vi "Test_Lockin_API.vi"() -> ()   [LabVIEW 2016]
uses:
  RemoteControl/Typedefs/Remote-SMO-Commands-Enum.ctl
  Typedefs/AO-cluster.ctl
  Typedefs/AO_Amp-array.ctl
  Typedefs/AO_DC-array.ctl
  Typedefs/AO_f-array.ctl
  Typedefs/AO_phi-array.ctl
  Typedefs/Function-array.ctl
  Typedefs/Function-enum.ctl
  Typedefs/REF-cluster.ctl
  Typedefs/REF_f-array.ctl
  Typedefs/REF_phi-array.ctl
  RemoteControl/RemoteControl.lvclass
panel:
  in  "Tab Control":enum32{"getResults", "getAO", "getAI", "config"}(tab)
  out "getResults":dbl(graph)
  in  "disabled index (col)":i32
  in  "disabled index (row)":i32
  out "getAO":waveform(dbl)[](graph)
  out "getAI":waveform(dbl)[](graph)
  in  "Channels: AO":T1 {"AO f (Hz)" min=0.001 max=10000.0; "AO DC (V)" format="%#_6p"; "AO amp (V)" format="%#_6p"}
  in  "Channels: Lockin":T8 {"REF phi (deg)" format="%#_3g"}
  in  "IV mode":bool
  in  "Remote Mode":bool=TRUE
  in  "Trigger":bool=TRUE
  out "ms watiing for IV curve":u32
  out "Numeric":i32
  in  "address":string
  in  "Enum":T11
  in  "Stop":bool
  # "0"
  # "1"
  # "2"
  # "3"
  # "4"
  # "5"
  # "6"
  # "7"
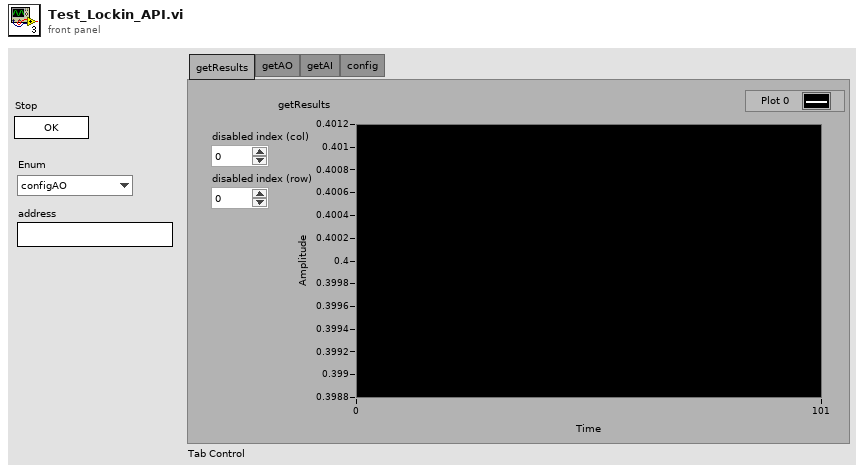
[diagram p1: front panel]
types:
  T1 = typedef "AO-cluster.ctl" = cluster{"AO amp (V)":T2, "AO DC (V)":T3, "AO f (Hz)":T4, "AO phi (deg)":T5, "function":T6}
  T2 = typedef "AO_Amp-array.ctl" = dbl[]
  T3 = typedef "AO_DC-array.ctl" = dbl[]
  T4 = typedef "AO_f-array.ctl" = dbl[]
  T5 = typedef "AO_phi-array.ctl" = dbl[]
  T6 = typedef "Function-array.ctl" = T7[]
  T7 = typedef "Function-enum.ctl" = enum16{"Sine Wave", "Triangle Wave", "Square Wave", "Sawtooth Wave"}
  T8 = typedef "REF-cluster.ctl" = cluster{"REF f (Hz)":T9, "REF phi (deg)":T10}
  T9 = typedef "REF_f-array.ctl" = dbl[]
  T10 = typedef "REF_phi-array.ctl" = dbl[]
  T11 = typedef "RemoteControl.lvclass/Remote-SMO-Commands-Enum.ctl" = enum16{"configAO", "configREF", "configIVmode", "configRemote", "assertTrigger", "getAO", "getAI", "getResults", "getTrigger", "getAOconfig", "getREFconfig", "ACK", "UNK", "CLOSE"}
  T12 = enum32{"invalid app kind", "Development System", "Run Time System", "Student Edition", "Embedded LabVIEW", "Evaluation", "Custom"}
  T13 = enum32{"Invalid", "Standard", "Closed", "Hidden", "Minimized", "Maximized"}
  T14 = cluster{"Core":cluster{"Current VI Reference":refnum<vi>, "Close Panel on Exit?":bool}, "Your Boolean data":bool, "remote address":string}
  T15 = cluster{"Current VI Reference":refnum<vi>, "Close Panel on Exit?":bool}
  T16 = typedef "RemoteControl.lvclass/PrivateEvents--RemoteControl.setTrigger.ctl" = bool
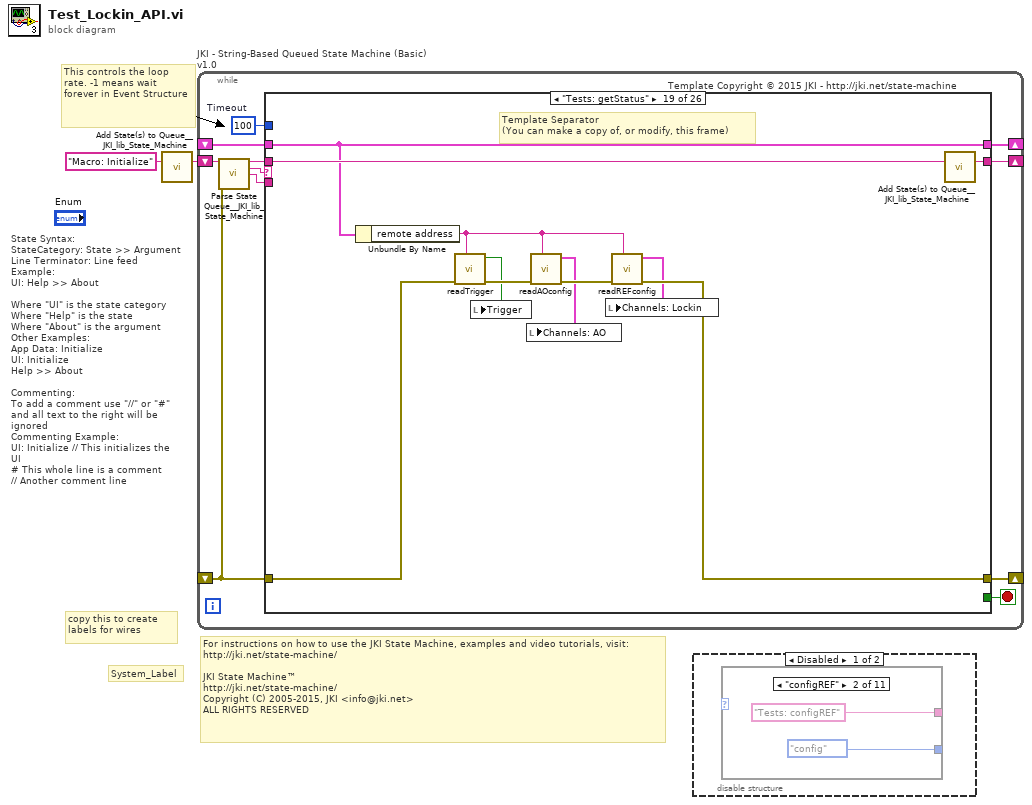
[diagram p0: block diagram]
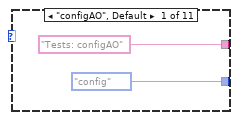
[diagram p2: hidden frame]
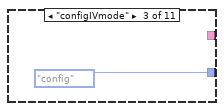
[diagram p3: hidden frame]
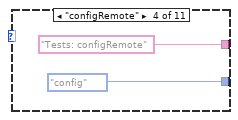
[diagram p4: hidden frame]
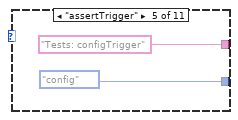
[diagram p5: hidden frame]
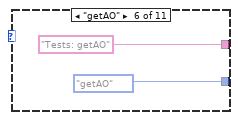
[diagram p6: hidden frame]
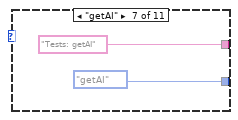
[diagram p7: hidden frame]
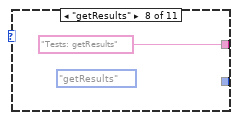
[diagram p8: hidden frame]
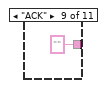
[diagram p9: hidden frame]
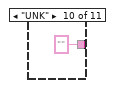
[diagram p10: hidden frame]
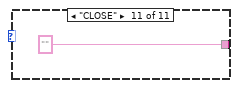
[diagram p11: hidden frame]
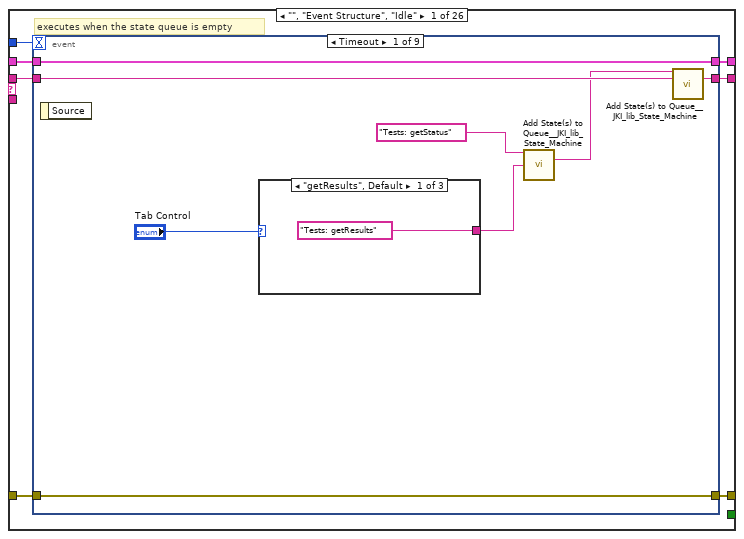
[diagram p13: hidden frame]
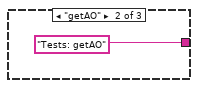
[diagram p14: hidden frame]
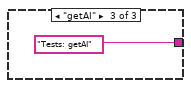
[diagram p15: hidden frame]
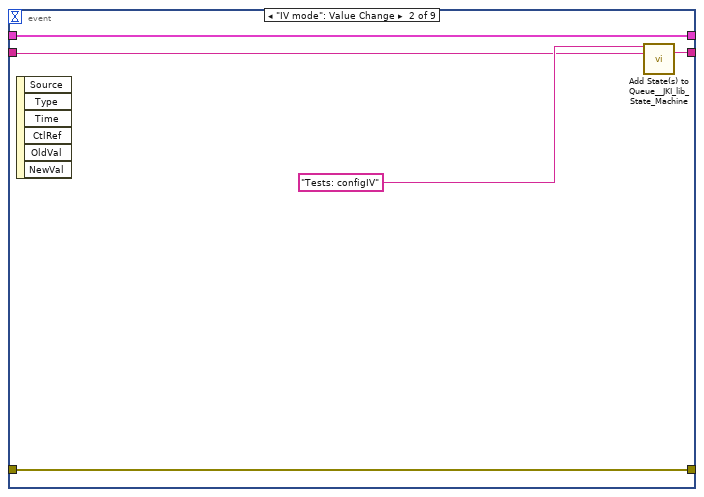
[diagram p16: hidden frame]
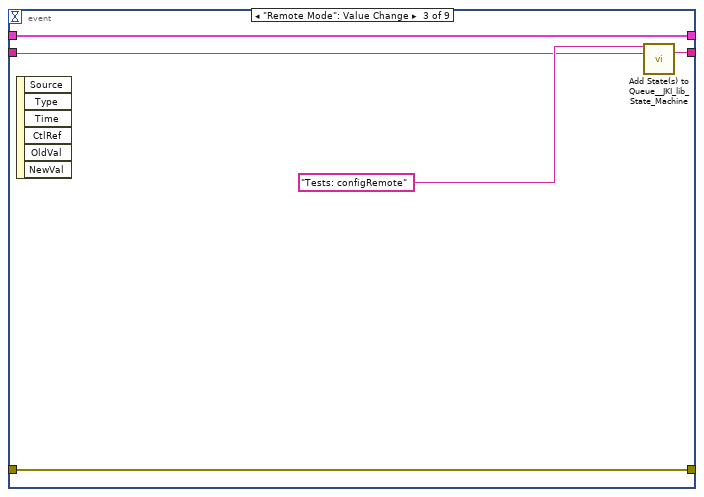
[diagram p17: hidden frame]
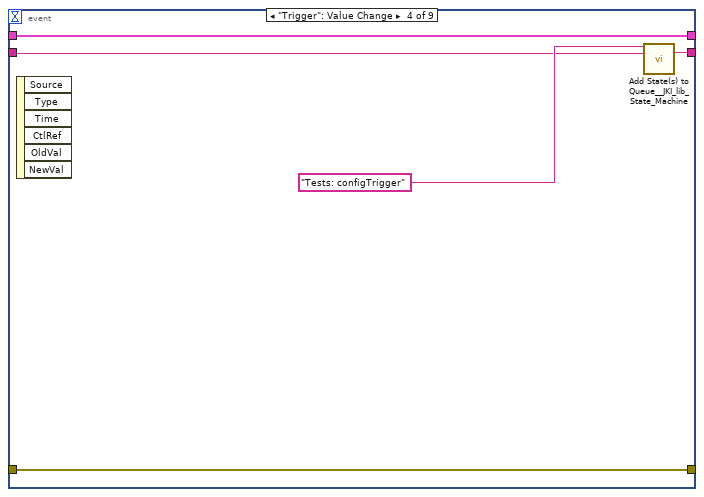
[diagram p18: hidden frame]
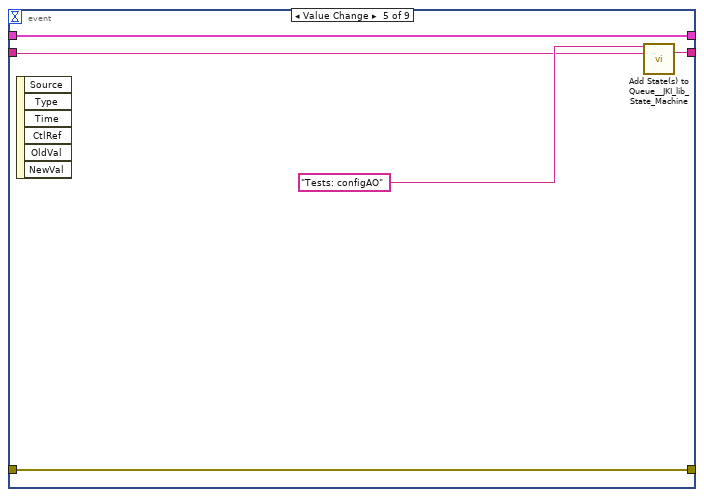
[diagram p19: hidden frame]
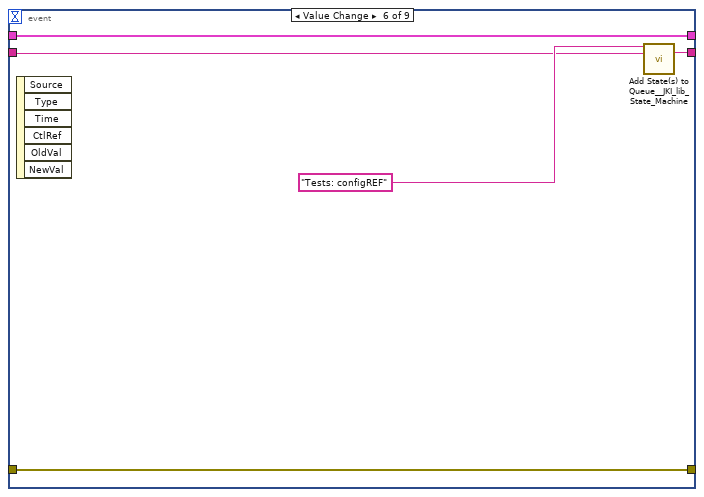
[diagram p20: hidden frame]
diagram:
  # "For instructions on how to use the JKI State Machine, examples and video tutorials, visit:\nhttp://jki.net/state-machine/\n\nJKI State Machine™\nhttp://jki.net/state-machine/\nCopyright (C) 2005-2015, JKI <info@jki.net>\nALL RIGHTS RESERVED"
  # "State Syntax:\nStateCategory: State >> Argument\nLine Terminator: Line feed\nExample:\nUI: Help >> About\n\nWhere \"UI\" is the state category\nWhere \"Help\" is the state\nWhere \"About\" is the argument\nOther Examples:\nApp Data: Initialize\nUI: Initialize\nHelp >> About\n\nCommenting:\nTo add a comment use \"//\" or \"#\" and all text to the right will be ignored\nCommenting Example:\nUI: Initialize // This initializes the UI\n# This whole line is a comment\n// Another comment line"
  # "copy this to create labels for wires"
  # "This controls the loop rate. -1 means wait forever in Event Structure"
  # "System_Label"
  n1 = call <vilib>:"Add State(s) to Queue__JKI_lib_State_Machine.vi"("State(s) in (\"\")"="Macro: Initialize") -> ("States Out"=w2:string)  [unwired: 14 in]
  n2 = while "JKI - String-Based Queued State Machine (Basic) v1.0" {
    shift-right: [w6] -> _
    shift-left: _ -> [w5]
    shift-right: [w9] -> _
    shift-left: _ -> [w3]
    shift-right: [w8] -> _
    shift-left: w2 -> [w10]
    stop <- w7 stop-if-true
    w4 = 100  # Timeout
    # "Template Copyright © 2015 JKI - http://jki.net/state-machine"
    n3 = call <vilib>:"Parse State Queue__JKI_lib_State_Machine.vi"("State Queue"=w10, "Error In (no error)"=w3) -> ("Remaining States"=w12:string, "Current State"=w13:string, "Arguments"=w11:string)  [unwired: 11 in]
    n4 = case shown="\"Tests: getStatus\"" w13 {
      selector: w13 -> [_ _ w78 _ _ _ _ _ _ _ _ _ _ _ _ _ _ _ _ _ _ _ _ _ _ _]
      tunnel: w12 -> [w20 w77 w82 w100 w106 w111 w115 w122 w128 w132 w136 w142 w153 w179 w184 w194 w198 w208 w219 w226 w233 w240 w247 w254 w261 w271]
      tunnel: w11 -> [_ _ _ _ _ _ _ _ _ _ _ w137 w147 _ _ _ _ _ _ _ _ _ _ _ _ _]
      tunnel: w5 -> [w18 w74 w80 w91 w103 w109 w112 _ w123 w129 w134 w140 w149 w176 w181 w191 w195 w200 w217 w220 w227 w234 w241 w248 w255 w266]
      tunnel: [w17 w75 w84 w97 errorcluster {"status"=FALSE, "code"=0, "source"=""} ("error out") w108 w113 w119 w124 w130 w133 w138 w150 w177 w182 w192 w196 w201 w212 w222 w230 w236 w243 w251 w258 w265] -> w9
      tunnel: w3 -> [w16 w75 w83 w97 w102 w108 w113 w119 w125 w130 w133 w139 w151 w177 w182 w192 w196 w202 w213 w224 w231 w237 w244 w252 w259 w269]
      tunnel: [w19 w76 w81 w99 w105 w110 w114 w121 w127 w131 w135 w141 w152 w178 w183 w193 w197 w207 w218 w225 w232 w239 w246 w253 w260 w270] -> w8
      tunnel: [_ _ _ _ _ TRUE _ _ _ _ _ _ _ _ _ _ _ _ _ _ _ _ _ _ _ _] -> w7
      tunnel: [w15 w74 w80 w98 w103 w109 w112 w120 w123 w129 w134 w140 w149 w176 w181 w191 w195 w200 w217 w220 w227 w234 w241 w248 w255 w266] -> w6
      tunnel: w4 -> [w14 _ _ _ _ _ _ _ _ _ _ _ _ _ _ _ _ _ _ _ _ _ _ _ _ _]
      frame "", "Event Structure", "Idle" {
        # "executes when the state queue is empty"
        n5 = event shown="[0] Timeout" {
          selector: _ -> [_ _ _ _ _ _ _ _ _]
          dyn-events: _ -> [_ _ _ _ _ _ _ _ _]
          timeout: w14 -> [_ _ _ _ _ _ _ _ _]
          tunnel: w20 -> [w28 w32 w37 w42 w47 w52 w61 w67 w73]
          tunnel: [w27 w36 w41 w46 w51 w56 w62 w66 w72] -> w19
          tunnel: w18 -> [w26 w33 w38 w43 w48 w53 w59 w64 w70]
          tunnel: [w24 w34 w39 w44 w49 w54 w60 w65 w71] -> w17
          tunnel: w16 -> [w24 w34 w39 w44 w49 w54 w60 w65 w71]
          tunnel: [w26 w33 w38 w43 w48 w53 w58 w64 w70] -> w15
          event Timeout {
            n6 = event-data() -> ()  [unwired: 1 in, 1 out]
            n7 = case shown="\"getResults\", Default" "Tab Control" {
              tunnel: ["Tests: getResults" "Tests: getAO" "Tests: getAI"] -> w23
              frame "getResults", Default {
              }
              frame "getAO" {
              }
              frame "getAI" {
              }
            }
            n8 = call <vilib>:"Add State(s) to Queue__JKI_lib_State_Machine.vi"("State(s) in Front (\"\")"="Tests: getStatus", "State(s) at Back (\"\")"=w23) -> ("States Out"=w22:string)  [unwired: 13 in]
            n9 = call <vilib>:"Add State(s) to Queue__JKI_lib_State_Machine.vi"("State(s) in Front (\"\")"=w22, "State(s) in (\"\")"=w28) -> ("States Out"=w27:string)  [unwired: 13 in]
          }
          event "IV mode": Value Change {
            n10 = event-data() -> ()  [unwired: 1 in, 6 out]
            n11 = call <vilib>:"Add State(s) to Queue__JKI_lib_State_Machine.vi"("State(s) in Front (\"\")"="Tests: configIV", "State(s) in (\"\")"=w32) -> ("States Out"=w36:string)  [unwired: 13 in]
          }
          event "Remote Mode": Value Change {
            n12 = event-data() -> ()  [unwired: 1 in, 6 out]
            n13 = call <vilib>:"Add State(s) to Queue__JKI_lib_State_Machine.vi"("State(s) in Front (\"\")"="Tests: configRemote", "State(s) in (\"\")"=w37) -> ("States Out"=w41:string)  [unwired: 13 in]
          }
          event "Trigger": Value Change {
            n14 = event-data() -> ()  [unwired: 1 in, 6 out]
            n15 = call <vilib>:"Add State(s) to Queue__JKI_lib_State_Machine.vi"("State(s) in Front (\"\")"="Tests: configTrigger", "State(s) in (\"\")"=w42) -> ("States Out"=w46:string)  [unwired: 13 in]
          }
          event Value Change {
            n16 = event-data() -> ()  [unwired: 1 in, 6 out]
            n17 = call <vilib>:"Add State(s) to Queue__JKI_lib_State_Machine.vi"("State(s) in Front (\"\")"="Tests: configAO", "State(s) in (\"\")"=w47) -> ("States Out"=w51:string)  [unwired: 13 in]
          }
          event Value Change {
            n18 = event-data() -> ()  [unwired: 1 in, 6 out]
            n19 = call <vilib>:"Add State(s) to Queue__JKI_lib_State_Machine.vi"("State(s) in Front (\"\")"="Tests: configREF", "State(s) in (\"\")"=w52) -> ("States Out"=w56:string)  [unwired: 13 in]
          }
          event "address": Value Change {
            n20 = event-data() -> ()  [unwired: 1 in, 6 out]
            n21 = Bundle By Name(cluster=w59, "remote address"="address") -> (w58:T14)
            n22 = call <vilib>:"Add State(s) to Queue__JKI_lib_State_Machine.vi"("State(s) in (\"\")"=w61) -> ("States Out"=w62:string)  [unwired: 14 in]
          }
          event "Stop": Value Change {
            # "Exit Button Value Change (pressed) Event\n(this executes Macro: Exit to terminate the VI)"
            n23 = event-data() -> ()  [unwired: 1 in, 1 out]
            n24 = call <vilib>:"Add State(s) to Queue__JKI_lib_State_Machine.vi"("State(s) in Front (\"\")"="Macro: Exit", "State(s) in (\"\")"=w67) -> ("States Out"=w66:string)  [unwired: 13 in]
          }
          event Panel Close? {
            # "Discard the event because we'll close the front panel ourselves in Macro: Exit"
            # "Close Panel button (pressed) Event\n(this executes Macro: Exit to terminate the VI)"
            n25 = event-data() -> ()  [unwired: 1 in, 1 out]
            n26 = event-data("Discard?"=TRUE) -> ()  [unwired: 1 in, 1 out]
            n27 = call <vilib>:"Add State(s) to Queue__JKI_lib_State_Machine.vi"("State(s) in Front (\"\")"="Macro: Exit", "State(s) in (\"\")"=w73) -> ("States Out"=w72:string)  [unwired: 13 in]
          }
        }
      }
      frame "---------- Core ----------" {
        # "Do not put any code in this frame.\n(it is a separator no-op)"
        n28 = call <vilib>:"Add State(s) to Queue__JKI_lib_State_Machine.vi"("State(s) in (\"\")"=w77) -> ("States Out"=w76:string)  [unwired: 14 in]
      }
      frame Default {
        w87 = 42 items=["No error", "Argument error", "Memory is full", "Out of zone", "End of file", "File already open", "Generic file I/O error", "File not found", "File permission error", "Disk is full", "Duplicate path", "Too many files open", "System feature not enabled", "Resource file not found", "Cannot add resource", "Resource not found", "Image not found", "Image memory error", "Pen does not exist", "Config type invalid", "Config token not found", "Config parse error", "Config memory error", "Bad external code format", "Bad external code offset", "External code not present", "Null window", "Destroy window error", "Null menu", "Print aborted", "Bad print record", "Print driver error", "Windows error during printing", "Memory error during printing", "Print dialog error", "Generic print error", "Invalid device refnum", "Device not found", "Device parameter error", "Device unit error", "Cannot open device", "Device call aborted", "Generic error", "Cancelled by user", "Object ID too low", "Object ID too high", "Object not in heap", "Unknown heap", "Unknown object (invalid DefProc)", "Unknown object (DefProc not in table)", "Message out of range", "Invalid (null) method", "Unknown message", "Manager call not supported", "Bad address", "Network operation in progress", "Network operation timed out", "Connection is busy", "Network attribute not supported", "Network error", "Address in use", "System out of memory", "Connection aborted", "Connection refused", "Not connected", "Already connected", "Connection closed", "Initialization error (interapplication manager)", "Bad occurrence", "Wait on unbound occurrence handler", "Occurrence queue overflow", "Datalog type conflict", "Unused", "Unrecognized type (interapplication manager)", "Memory corrupt", "Failed to make temporary DLL", "Old CIN version", "Drag socket not found", "Failed to load drop-object", "Failed to register OLE object", "Failed to release OLE object", "Format specifier type mismatch", "Unknown format specifier", "Too few format specifiers", "Too many format specifiers", "Scan failed", "Newer CIN version", "Error converting to variant", "Runtime menu error", "Password tampered", "Variant attribute not found", "Incompatible variant data type", "Event data is not available", "Event Store is not present", "Occurrence is not found", "Event Queue is not created", "Event info is not available", "Refnum passed is NULL", "Error retrieving Class GUID", "Error retrieving CoClass GUID", "Error retrieving TypeLib GUID.", "Bad built application magic bytes.", "Specific driver is different from the specific driver associated with the Logical Name.", "There is no session opened to the class driver.", "Max Error", "MAX - Error with config objects", "MAX - Error loading configuration", "MAX - Group not supported"]
        # "Current State"
        # "Do not delete, rename, or modify this frame.\n(this is used to capture unhandled states and typos)"
        # "Handle mistyped state name (developer tool)"
        n29 = Format Into String(format string="Software Exception: Unhandled State \"%s\"." ("message"), error in=w83, w78) -> (resulting string=w86:string, error out=w85:errorcluster)  [unwired: 1 in]
        n30 = call <vilib>:"Error Cluster From Error Code.vi"("show call chain? (False)"=TRUE, "error in (no error)"=w85, "error message (\"\")"=w86, "error code (0)"=w87) -> ("error out"=w84:errorcluster)  [unwired: 5 in]
        n31 = call <vilib>:"Add State(s) to Queue__JKI_lib_State_Machine.vi"("State(s) in (\"\")"=w82) -> ("States Out"=w81:string)  [unwired: 14 in]
      }
      frame "Initialize Core Data" {
        # "Do not delete, rename, or modify this frame.\n(this is used to determine panel behavior on exit)"
        # "originally closed?"
        # "exe?"
        # "If panel starts closed or is an EXE, then close it when we exit"
        n32 = property class="VI"() -> ("Front Panel.Open"=w96:bool)  [unwired: 2 in, 2 out]
        n33 = property class="App"() -> ("App.Kind"=w95:T12)  [unwired: 2 in, 2 out]
        n34 = control-ref of="Current VI Reference"() -> (w89:refnum<vi>)
        n35 = Not(x=w96) -> (.not. x?=w93:bool)
        n36 = Equal?(x=w95, y=T12."Run Time System" ("Application:Kind")) -> (x = y?=w92:bool)
        n37 = Or(x=w93, y=w92) -> (x .or. y?=w90:bool)
        n38 = Bundle By Name(cluster=w91, "Core.Current VI Reference"=w89, "Core.Close Panel on Exit?"=w90) -> (w98:T14)
        n39 = call <vilib>:"Add State(s) to Queue__JKI_lib_State_Machine.vi"("State(s) in (\"\")"=w100) -> ("States Out"=w99:string)  [unwired: 14 in]
      }
      frame "Error Handler" {
        # "Unhandled Error -- Display it"
        # "Handle any errors here.\nYou can also output any states to clean-up after errors occur"
        # "Clear error"
        n40 = call <vilib>:"General Error Handler.vi"("error in (no error)"=w102) -> ()  [unwired: 10 in, 5 out]
        n41 = call <vilib>:"Add State(s) to Queue__JKI_lib_State_Machine.vi"("State(s) in Front (\"\")"="/* Post Error States", "State(s) in (\"\")"=w106) -> ("States Out"=w105:string)  [unwired: 13 in]
      }
      frame "Exit" {
        # "Do not put any code in this frame.\n(No errors that occur here will be handled.)"
        n42 = call <vilib>:"Add State(s) to Queue__JKI_lib_State_Machine.vi"("State(s) in (\"\")"=w111) -> ("States Out"=w110:string)  [unwired: 14 in]
      }
      frame "---------- Data ----------" {
        # "Do not put any code in this frame.\n(It is a separator no-op. You can make a copy of this frame to create a new Data frame)"
        n43 = call <vilib>:"Add State(s) to Queue__JKI_lib_State_Machine.vi"("State(s) in (\"\")"=w115) -> ("States Out"=w114:string)  [unwired: 14 in]
      }
      frame "Data: Initialize" {
        w116 = T15 {"Current VI Reference"=refnum, "Close Panel on Exit?"=FALSE}  # Core
        w118 = TRUE  # Your Boolean data
        w117 = ""  # remote address
        # "do not delete - used by framework"
        # "Expand Bundle to add new data elements to shift register data."
        # "Data names and types of shift register data are defined by this bundle."
        # "Initialize the shift-register data, here.\n(data names are defined by what you wire into the bundle function)"
        n44 = Bundle("Core"=w116, "Your Boolean data"=w118, "remote address"=w117) -> (w120:T14)  [unwired: 1 in]
        n45 = call <vilib>:"Add State(s) to Queue__JKI_lib_State_Machine.vi"("State(s) in (\"\")"=w122) -> ("States Out"=w121:string)  [unwired: 14 in]
      }
      frame "Data: Cleanup" {
        # "Cleanup any data and references, here.\n(this is called automatically, by the Macro: Exit)"
        n46 = Unbundle By Name(w123) -> ("Core.Current VI Reference"=w126:refnum<vi>)
        n47 = Close Reference(reference=w126, error in (no error)=w125) -> (error out=w124:errorcluster)
        n48 = call <vilib>:"Add State(s) to Queue__JKI_lib_State_Machine.vi"("State(s) in (\"\")"=w128) -> ("States Out"=w127:string)  [unwired: 14 in]
      }
      frame "---------- UI ----------" {
        # "Do not put any code in this frame.\n(It is a separator no-op. You can make a copy of this frame to create a new UI frame)"
        n49 = call <vilib>:"Add State(s) to Queue__JKI_lib_State_Machine.vi"("State(s) in (\"\")"=w132) -> ("States Out"=w131:string)  [unwired: 14 in]
      }
      frame "UI: Initialize" {
        # "Initialize the User Interface, here.\n(this is called automatically, by the Macro: Init)"
        n50 = call <vilib>:"Add State(s) to Queue__JKI_lib_State_Machine.vi"("State(s) in (\"\")"=w136) -> ("States Out"=w135:string)  [unwired: 14 in]
      }
      frame "UI: Cursor Set" {
        # "Argument"
        # "Set and Unset Cursor Busy.\n(Usage: \"UI: Cursor Set >> Busy|Idle\")"
        n51 = case shown="\"Idle\", Default" w137 {
          tunnel: w139 -> [w144 w146]
          tunnel: [w143 w145] -> w138
          frame "Idle", Default {
            n52 = call <vilib>:"Unset Busy.vi"("error in (no error)"=w144) -> ("error out"=w143:errorcluster)  [unwired: 10 in]
          }
          frame "Busy" {
            n53 = call <vilib>:"Set Busy.vi"("error in (no error)"=w146) -> ("error out"=w145:errorcluster)  [unwired: 9 in, 1 out]
          }
        }
        n54 = call <vilib>:"Add State(s) to Queue__JKI_lib_State_Machine.vi"("State(s) in (\"\")"=w142) -> ("States Out"=w141:string)  [unwired: 14 in]
      }
      frame "UI: Front Panel State" {
        # "Argument"
        # "Set Front Panel Open or Closed\n(Usage: \"UI: Front Panel State >> Open|Close\")"
        n55 = Unbundle By Name(w149) -> ("Core.Current VI Reference"=w148:refnum<vi>)
        n56 = case shown="\"Open\", Default" w147 {
          tunnel: w151 -> [w157 w170]
          tunnel: [w159 w171] -> w150
          tunnel: w148 -> [w158 w168]
          frame "Open", Default {
            n57 = property class="VI"(reference=w158, error in=w157) -> (reference out=w155:refnum<vi>, error out=w156:errorcluster, "Front Panel.Open"=w154:bool)
            n58 = case shown="False" w154 {
              tunnel: [w162 w165] -> w159
              tunnel: w156 -> [w161 w165]
              tunnel: w155 -> [w160 _]
              frame False {
                n59 = invoke class="VI" method="FP.Open"(reference=w160, error in=w161, "Activate"=TRUE, "State"=T13."Standard") -> (error out=w162:errorcluster)  [unwired: 1 in, 4 out]
              }
              frame True {
              }
            }
          }
          frame "Close" {
            n60 = property class="VI"(reference=w168, error in=w170) -> (reference out=w167:refnum<vi>, error out=w169:errorcluster, "Front Panel.Open"=w166:bool)
            n61 = case shown="True" w166 {
              tunnel: [w172 w175] -> w171
              tunnel: w169 -> [w172 w174]
              tunnel: w167 -> [_ w173]
              frame False {
              }
              frame True {
                n62 = invoke class="VI" method="FP.Close"(reference=w173, error in=w174) -> (error out=w175:errorcluster)  [unwired: 1 in, 2 out]
              }
            }
          }
        }
        n63 = call <vilib>:"Add State(s) to Queue__JKI_lib_State_Machine.vi"("State(s) in (\"\")"=w153) -> ("States Out"=w152:string)  [unwired: 14 in]
      }
      frame "---------- Macro ----------" {
        # "Do not put any code in this frame.\n(It is a separator no-op. You can make a copy of this frame to create a new Macro frame)"
        n64 = call <vilib>:"Add State(s) to Queue__JKI_lib_State_Machine.vi"("State(s) in (\"\")"=w179) -> ("States Out"=w178:string)  [unwired: 14 in]
      }
      frame "Macro: Initialize" {
        w180 = "Data: Initialize\nInitialize Core Data\nUI: Initialize\nUI: Front Panel State >> Open"  # Data: Initialize Initialize Core Data UI: Initialize UI: Front Panel State >> Open
        # "Initialization Macro\n(This is called once, when the VI starts)"
        n65 = call <vilib>:"Add State(s) to Queue__JKI_lib_State_Machine.vi"("State(s) in Front (\"\")"=w180, "State(s) in (\"\")"=w184) -> ("States Out"=w183:string)  [unwired: 13 in]
      }
      frame "Macro: Exit" {
        # "Exit Macro\n(This is called once, when the VI exits)"
        n66 = Unbundle By Name(w191) -> ("Core.Close Panel on Exit?"=w190:bool)
        n67 = Select(t="UI: Front Panel State >> Close", s=w190, f="") -> (s? t:f=w187:string)
        n68 = call <vilib>:"Add State(s) to Queue__JKI_lib_State_Machine.vi"("State(s) in (\"\")"=w187, "State(s) at Back (\"\")"="Data: Cleanup\nExit") -> ("States Out"=w185:string)  [unwired: 13 in]
        n69 = call <vilib>:"Add State(s) to Queue__JKI_lib_State_Machine.vi"("State(s) in Front (\"\")"=w185, "State(s) in (\"\")"=w194) -> ("States Out"=w193:string)  [unwired: 13 in]
      }
      frame "---------- Tests ----------" {
        # "Template Separator\n(You can make a copy of, or modify, this frame)"
        n70 = call <vilib>:"Add State(s) to Queue__JKI_lib_State_Machine.vi"("State(s) in (\"\")"=w198) -> ("States Out"=w197:string)  [unwired: 14 in]
      }
      frame "Tests: getResults" {
        n71 = Unbundle By Name(w200) -> ("remote address"=w199:string)
        n72 = call "readResults.vi"("address"=w199, "error in (no error)"=w202) -> ("error out"=w201:errorcluster, "Results"=w203:dbl[][])  [unwired: 8 in]
        n73 = Index Array(array=w203, index (row)="disabled index (row)", index (col)="disabled index (col)") -> (element=→"getResults":dbl)
        n74 = call <vilib>:"Add State(s) to Queue__JKI_lib_State_Machine.vi"("State(s) in (\"\")"=w208) -> ("States Out"=w207:string)  [unwired: 14 in]
      }
      frame "Tests: getStatus" {
        # "Template Separator\n(You can make a copy of, or modify, this frame)"
        n75 = Unbundle By Name(w217) -> ("remote address"=w216:string)
        n76 = call "readTrigger.vi"("address"=w216, "error in (no error)"=w213) -> ("error out"=w215:errorcluster, "Trigger"=w209:T16)  [unwired: 8 in]
        n77 = local write "Trigger"(w209) -> ()
        n78 = call "readAOconfig.vi"("address"=w216, "error in (no error)"=w215) -> ("error out"=w214:errorcluster, "AOconfig"=w211:T1)  [unwired: 8 in]
        n79 = local write "Channels: AO"(w211) -> ()
        n80 = call "readREFconfig.vi"("address"=w216, "error in (no error)"=w214) -> ("error out"=w212:errorcluster, "REFconfig"=w210:T8)  [unwired: 8 in]
        n81 = local write "Channels: Lockin"(w210) -> ()
        n82 = call <vilib>:"Add State(s) to Queue__JKI_lib_State_Machine.vi"("State(s) in (\"\")"=w219) -> ("States Out"=w218:string)  [unwired: 14 in]
      }
      frame "Tests: getAI" {
        n83 = Unbundle By Name(w220) -> ("remote address"=w221:string)
        n84 = call "readAI.vi"("address"=w221, "error in (no error)"=w224) -> ("error out"=w222:errorcluster, "input signal"=→"getAI":waveform(dbl)[])  [unwired: 8 in]
        n85 = call <vilib>:"Add State(s) to Queue__JKI_lib_State_Machine.vi"("State(s) in (\"\")"=w226) -> ("States Out"=w225:string)  [unwired: 14 in]
      }
      frame "Tests: getAO" {
        n86 = Unbundle By Name(w227) -> ("remote address"=w228:string)
        n87 = call "readAO.vi"("address"=w228, "error in (no error)"=w231) -> ("error out"=w230:errorcluster, "output signal"=→"getAO":waveform(dbl)[])  [unwired: 8 in]
        n88 = call <vilib>:"Add State(s) to Queue__JKI_lib_State_Machine.vi"("State(s) in (\"\")"=w233) -> ("States Out"=w232:string)  [unwired: 14 in]
      }
      frame "Tests: configAO" {
        n89 = Unbundle By Name(w234) -> ("remote address"=w235:string)
        n90 = call "configAO.vi"("address"=w235, "error in (no error)"=w237, "Channels: AO in"="Channels: AO") -> ("error out"=w236:errorcluster)  [unwired: 7 in, 1 out]
        n91 = call <vilib>:"Add State(s) to Queue__JKI_lib_State_Machine.vi"("State(s) in (\"\")"=w240) -> ("States Out"=w239:string)  [unwired: 14 in]
      }
      frame "Tests: configREF" {
        n92 = Unbundle By Name(w241) -> ("remote address"=w242:string)
        n93 = call "configREF.vi"("address"=w242, "error in (no error)"=w244, "Channels: Lockin in"="Channels: Lockin") -> ("error out"=w243:errorcluster)  [unwired: 7 in, 1 out]
        n94 = call <vilib>:"Add State(s) to Queue__JKI_lib_State_Machine.vi"("State(s) in (\"\")"=w247) -> ("States Out"=w246:string)  [unwired: 14 in]
      }
      frame "Tests: configIV" {
        n95 = Unbundle By Name(w248) -> ("remote address"=w249:string)
        n96 = call "configIVmode.vi"("address"=w249, "error in (no error)"=w252, "IV mode"="IV mode") -> ("error out"=w251:errorcluster)  [unwired: 8 in]
        n97 = call <vilib>:"Add State(s) to Queue__JKI_lib_State_Machine.vi"("State(s) in (\"\")"=w254) -> ("States Out"=w253:string)  [unwired: 14 in]
      }
      frame "Tests: configRemote" {
        n98 = Unbundle By Name(w255) -> ("remote address"=w256:string)
        n99 = call "configRemote.vi"("address"=w256, "error in (no error)"=w259, "Remote Mode"="Remote Mode") -> ("error out"=w258:errorcluster)  [unwired: 8 in]
        n100 = call <vilib>:"Add State(s) to Queue__JKI_lib_State_Machine.vi"("State(s) in (\"\")"=w261) -> ("States Out"=w260:string)  [unwired: 14 in]
      }
      frame "Tests: configTrigger" {
        n101 = Unbundle By Name(w266) -> ("remote address"=w267:string)
        n102 = call "assertTrigger.vi"("address"=w267, "error in (no error)"=w269, "Trigger"="Trigger") -> ("error out"=w263:errorcluster)  [unwired: 8 in]
        n103 = call <userlib>:"Tick Count (ms)__ogtk.vi"("error in (no error)"=w263) -> ("error out"=w264:errorcluster, "millisecond timer value"=w262:u32)  [unwired: 9 in]
        n104 = while {
          tunnel: w267 -> [w280]
          shift-right: [w279] -> w265
          shift-left: w264 -> [w277]
          tunnel: w262 -> [w275]
          i -> [w272]
          stop <- w273 continue-if-true
          n105 = call <userlib>:"Tick Count (ms)__ogtk.vi"("error in (no error)"=w277) -> ("error out"=w278:errorcluster, "millisecond timer value"=w276:u32)  [unwired: 9 in]
          n106 = Subtract(x=w276, y=w275) -> (x-y=→"ms watiing for IV curve":u32)
          n107 = call "readTrigger.vi"("address"=w280, "error in (no error)"=w278) -> ("error out"=w279:errorcluster, "Trigger"=w273:T16)  [unwired: 8 in]
          n108 = local write "Trigger"(w273) -> ()
          "Numeric" <- w272
        }
        n109 = call <vilib>:"Add State(s) to Queue__JKI_lib_State_Machine.vi"("State(s) in (\"\")"=w271) -> ("States Out"=w270:string)  [unwired: 14 in]
      }
    }
  }
  n110 = disable-structure shown="Disabled" {
    frame Disabled {
      n111 = case shown="\"configREF\"" {
        selector: _ -> [_ _ _ _ _ _ _ _ _ _ _]
        tunnel: ["Tests: configAO" "Tests: configREF" w286 "Tests: configRemote" "Tests: configTrigger" "Tests: getAO" "Tests: getAI" "Tests: getResults" "" "" ""] -> _
        tunnel: [enum32{"getResults", "getAO", "getAI", "config"}."config" ("Tab Control") enum32{"getResults", "getAO", "getAI", "config"}."config" ("Tab Control") enum32{"getResults", "getAO", "getAI", "config"}."config" ("Tab Control") enum32{"getResults", "getAO", "getAI", "config"}."config" ("Tab Control") enum32{"getResults", "getAO", "getAI", "config"}."config" ("Tab Control") enum32{"getResults", "getAO", "getAI", "config"}."getAO" ("Tab Control") enum32{"getResults", "getAO", "getAI", "config"}."getAI" ("Tab Control") _ _ _ _] -> _
        frame "configAO", Default {
        }
        frame "configREF" {
        }
        frame "configIVmode" {
        }
        frame "configRemote" {
        }
        frame "assertTrigger" {
        }
        frame "getAO" {
        }
        frame "getAI" {
        }
        frame "getResults" {
          (unwired) enum32{"getResults", "getAO", "getAI", "config"}."getResults" ("Tab Control")
        }
        frame "ACK" {
        }
        frame "UNK" {
        }
        frame "CLOSE" {
        }
      }
    }
    frame Enabled {
    }
  }
